vi "decode access token response.vi"(8 "error in (no error)":errorcluster, 9 "Response":string, 10 "Header":string, 11 "Oauth2 in":refnum<class "Oauth2.lvclass">) -> (0 "error out":errorcluster, 3 "Oauth2":refnum<class "Oauth2.lvclass">)   [LabVIEW 2020, in "Oauth2.lvclass"]
uses:
  Oauth2.lvclass
  OAuthToken/OAuth2 Token Element -- enum.ctl
  OAuthToken/OAuthAccessToken.lvclass
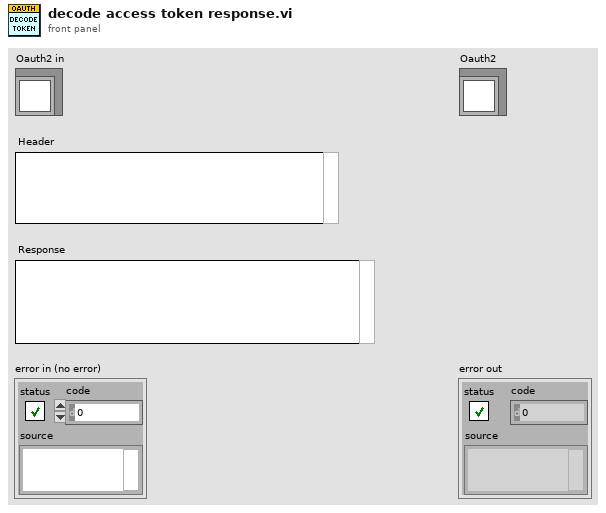
[diagram p1: front panel]
types:
  T1 = typedef "OAuthAccessToken.lvclass/OAuth2 Token Element -- enum.ctl" = enum16{"client_id", "client_secret", "response_type", "scope", "redirect_uri", "error", "error_description", "error_uri", "grant_type", "code", "access_token", "token_type", "expires_in", "username", "password", "refresh_token", "code_challenge", "code_challenge_method", "reverse_proxy_uri", "endpoint element"}
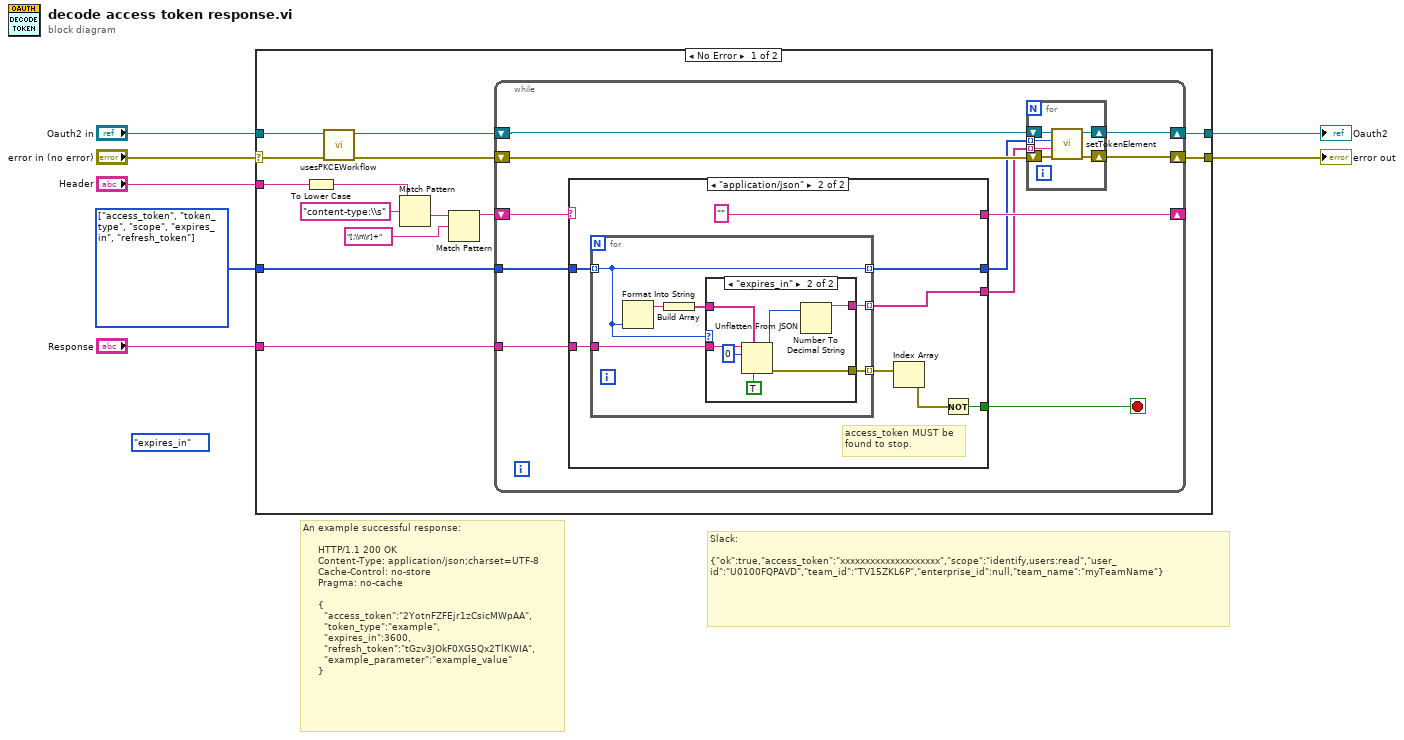
[diagram p0: block diagram]
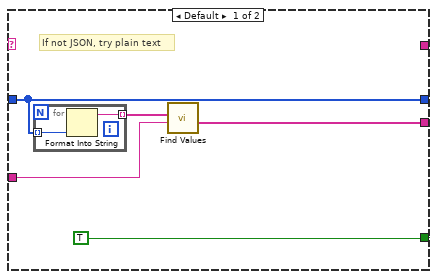
[diagram p2: hidden frame]
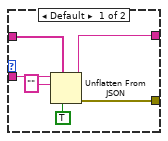
[diagram p3: hidden frame]
diagram:
  (unwired) OAuth2_Token_Element_--_enum."expires_in" ("Token element")
  w1 = T1[] [enum."access_token", enum."token_type", enum."scope", enum."expires_in", enum."refresh_token"] items=["client_id", "client_secret", "response_type", "scope", "redirect_uri", "error", "error_description", "error_uri", "grant_type", "code", "access_token", "token_type", "expires_in", "username", "password", "refresh_token", "code_challenge", "code_challenge_method", "reverse_proxy_uri", "endpoint element"]
  # "Slack:\n\n{\"ok\":true,\"access_token\":\"xxxxxxxxxxxxxxxxxxxx\",\"scope\":\"identify,users:read\",\"user_id\":\"U0100FQPAVD\",\"team_id\":\"TV15ZKL6P\",\"enterprise_id\":null,\"team_name\":\"myTeamName\"}"
  # "An example successful response:\n\n     HTTP/1.1 200 OK\n     Content-Type: application/json;charset=UTF-8\n     Cache-Control: no-store\n     Pragma: no-cache\n\n     {\n       \"access_token\":\"2YotnFZFEjr1zCsicMWpAA\",\n       \"token_type\":\"example\",\n       \"expires_in\":3600,\n       \"refresh_token\":\"tGzv3JOkF0XG5Qx2TlKWIA\",\n       \"example_parameter\":\"example_value\"\n     }"
  n1 = case shown="No Error" "error in (no error)" {
    selector: "error in (no error)" -> [w9 w74]
    tunnel: [w19 w74] -> w6
    tunnel: [w20 w73] -> w4
    tunnel: "Oauth2 in" -> [w11 w73]
    tunnel: "Response" -> [w21 _]
    tunnel: "Header" -> [w18 _]
    tunnel: w1 -> [w13 _]
    frame No Error {
      n2 = To Lower Case(string=w18) -> (all lower case string=w12:string)
      n3 = call "usesPKCEWorkflow.vi"("error in (no error)"=w9, "Oauth2 in"=w11) -> ("error out"=w8:errorcluster, "Oauth2 out"=w10:refnum<class "Oauth2.lvclass">)  [unwired: 7 in, 1 out]
      n4 = Match Pattern(string=w12, regular expression="content-type:\\s") -> (after substring=w16:string)  [unwired: 1 in, 3 out]
      n5 = Match Pattern(string=w16, regular expression="[;\\n\\r]+") -> (before substring=w14:string)  [unwired: 1 in, 3 out]
      n6 = while {
        tunnel: w21 -> [w32]
        shift-right: [w27] -> w20
        shift-left: w10 -> [w25]
        shift-right: [w26] -> w19
        shift-left: w8 -> [w24]
        shift-right: [w29] -> _
        shift-left: w14 -> [w30]
        tunnel: w13 -> [w28]
        stop <- w31 stop-if-true
        n7 = case shown="\"application/json\"" w30 {
          tunnel: w32 -> [w40 w53]
          tunnel: [TRUE w50] -> w31
          tunnel: [_ "" ("regular expression")] -> w29
          tunnel: w28 -> [w42 w48]
          tunnel: [w42 w47] -> w23
          tunnel: [w39 w46] -> w22
          frame Default {
            # "If not JSON, try plain text"
            n8 = for {
              tunnel: w42 -> [w45] mode=indexing
              tunnel: [w44] -> w41 mode=indexing
              n9 = Format Into String(w45) -> (resulting string=w44:string)  [unwired: 3 in, 1 out]
            }
            n10 = call "Find Values.vi"("Response string"=w40, "keys"=w41) -> ("values"=w39:string[])  [unwired: 8 in, 1 out]
          }
          frame "application/json" {
            # "access_token MUST be\nfound to stop."
            n11 = for {
              tunnel: w53 -> [w59]
              tunnel: [w58] -> w52 mode=indexing
              tunnel: w48 -> [w54] mode=indexing
              tunnel: [w54] -> w47 mode=indexing
              tunnel: [w56] -> w46 mode=indexing
              n12 = Format Into String(w54) -> (resulting string=w57:string)  [unwired: 3 in, 1 out]
              n13 = Build Array(w57) -> (w55:string[])
              n14 = case shown="\"expires_in\"" w54 {
                tunnel: w59 -> [w65 w72]
                tunnel: [w64 w71] -> w58
                tunnel: [w62 w67] -> w56
                tunnel: w55 -> [w61 w69]
                frame Default {
                  n15 = Unflatten From JSON(path=w61, JSON string=w65, type and defaults="", default null elements? (F)=TRUE) -> (value=w62:string, error out=w64:errorcluster)  [unwired: 3 in]
                }
                frame "expires_in" {
                  n16 = Unflatten From JSON(path=w69, JSON string=w72, type and defaults=u32 0, default null elements? (F)=TRUE) -> (value=w66:u32, error out=w71:errorcluster)  [unwired: 3 in]
                  n17 = Number To Decimal String(number=w66) -> (decimal integer string=w67:string)  [unwired: 1 in]
                }
              }
            }
            n18 = Index Array(array=w52) -> (element=w51:errorcluster)  [unwired: 1 in]
            n19 = Not(x=w51) -> (.not. x?=w50:bool)
          }
        }
        n20 = for {
          shift-right: [w37] -> w27
          shift-left: w25 -> [w38]
          shift-right: [w35] -> w26
          shift-left: w24 -> [w36]
          tunnel: w23 -> [w34] mode=indexing
          tunnel: w22 -> [w33] mode=indexing
          n21 = call "setTokenElement.vi"("error in (no error)"=w36, "Value"=w33, "Token element"=w34, "Oauth2 in"=w38) -> ("error out"=w35:errorcluster, "Oauth2 out"=w37:refnum<class "Oauth2.lvclass">)  [unwired: 6 in]
        }
      }
    }
    frame Error {
    }
  }
  "error out" <- w6
  "Oauth2" <- w4
